vi "test-AsyncMessageWithReplyWithErrorWithGlobalVariable.vi"(8 "error in (no error)":errorcluster, 11 "TestCase in":refnum<class "testcase-CSMMessage.lvclass">) -> (0 "error out":errorcluster, 3 "TestCase out":refnum<class "testcase-CSMMessage.lvclass">)   [LabVIEW 2017, in "testcase-CSMMessage.lvclass"]
uses:
  testcase-CSMMessage.lvclass
  C:/Program Files (x86)/National Instruments/LabVIEW 2017/vi.lib/addons/_JKI Toolkits/VI Tester/TestCase.llb/TestCase.lvclass
  src/user.lib/_NEVSTOP/Communicable State Machine(CSM)/Communicable State Machine.lvlib
  CSM/Global-TestcaseCSM.vi
  CSM/CSM-Testcase.lvlib
  <vilib>/addons/_JKI Toolkits/VI Tester/TestCase.llb/TestCase.lvclass
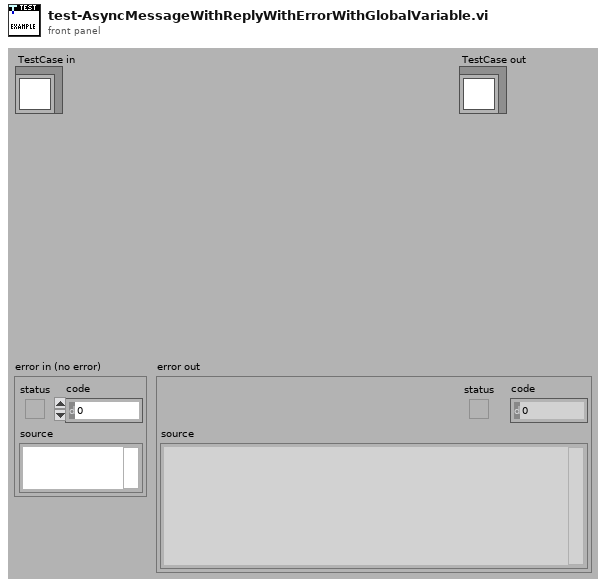
[diagram p1: front panel]
types:
  T1 = cluster{"Arguments":string, "Response":string, "error":errorcluster}
  T2 = cluster{"status":bool, "code":bool, "source":bool}
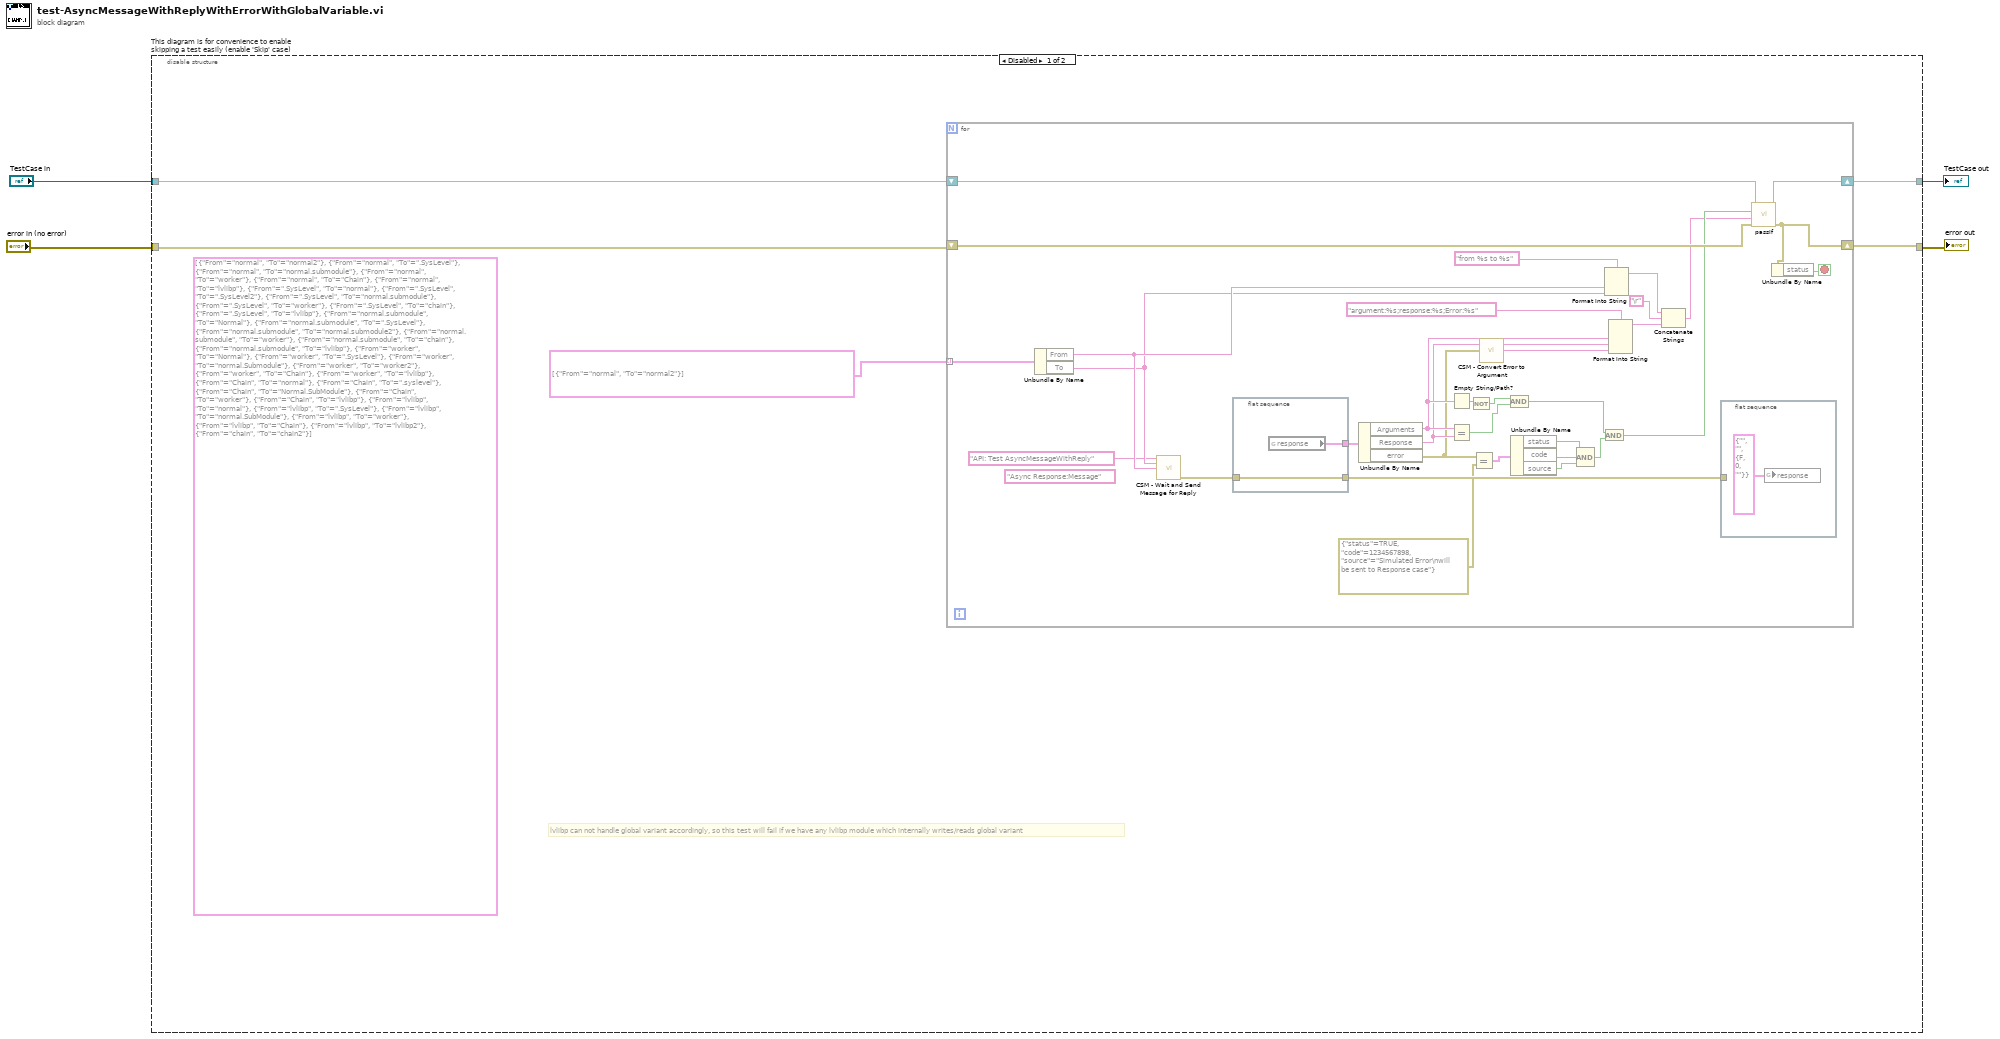
[diagram p0: block diagram]
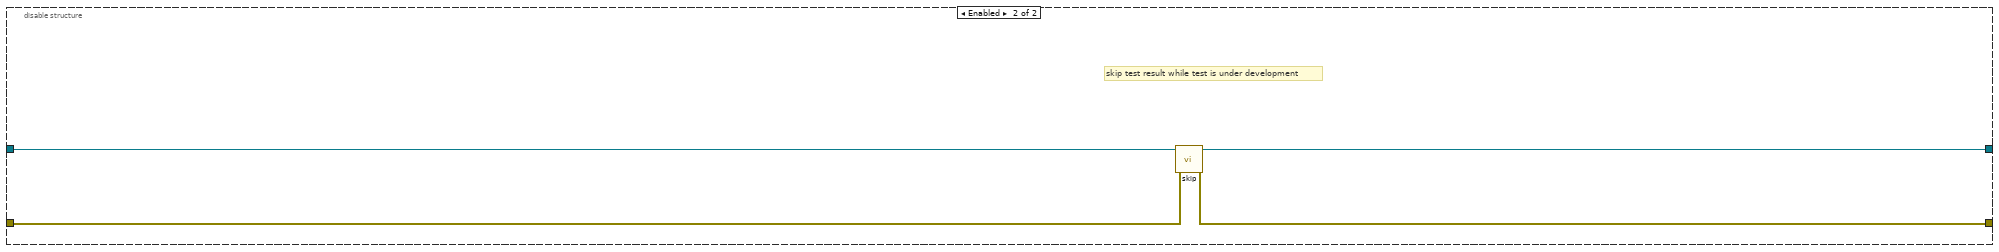
[diagram p2: hidden frame]
diagram:
  n1 = disable-structure "This diagram is for convenience to enable skipping a test easily (enable 'Skip' case)" shown="Disabled" {
    disable-tunnel: "TestCase in" -> [w9 w49]
    disable-tunnel: [w8 w47] -> w1
    disable-tunnel: [w6 w48] -> w3
    disable-tunnel: "error in (no error)" -> [w7 w46]
    frame Disabled {
      (unwired) cluster{"From":string, "To":string}[] [{"From"="normal", "To"="normal2"}, {"From"="normal", "To"=".SysLevel"}, {"From"="normal", "To"="normal.submodule"}, {"From"="normal", "To"="worker"}, {"From"="normal", "To"="Chain"}, {"From"="normal", "To"="lvlibp"}, {"From"=".SysLevel", "To"="normal"}, {"From"=".SysLevel", "To"=".SysLevel2"}, {"From"=".SysLevel", "To"="normal.submodule"}, {"From"=".SysLevel", "To"="worker"}, {"From"=".SysLevel", "To"="chain"}, {"From"=".SysLevel", "To"="lvlibp"}, {"From"="normal.submodule", "To"="Normal"}, {"From"="normal.submodule", "To"=".SysLevel"}, {"From"="normal.submodule", "To"="normal.submodule2"}, {"From"="normal.submodule", "To"="worker"}, {"From"="normal.submodule", "To"="chain"}, {"From"="normal.submodule", "To"="lvlibp"}, {"From"="worker", "To"="Normal"}, {"From"="worker", "To"=".SysLevel"}, {"From"="worker", "To"="normal.Submodule"}, {"From"="worker", "To"="worker2"}, {"From"="worker", "To"="Chain"}, {"From"="worker", "To"="lvlibp"}, {"From"="Chain", "To"="normal"}, {"From"="Chain", "To"=".syslevel"}, {"From"="Chain", "To"="Normal.SubModule"}, {"From"="Chain", "To"="worker"}, {"From"="Chain", "To"="lvlibp"}, {"From"="lvlibp", "To"="normal"}, {"From"="lvlibp", "To"=".SysLevel"}, {"From"="lvlibp", "To"="normal.SubModule"}, {"From"="lvlibp", "To"="worker"}, {"From"="lvlibp", "To"="Chain"}, {"From"="lvlibp", "To"="lvlibp2"}, {"From"="chain", "To"="chain2"}]
      # "lvlibp can not handle global variant accordingly, so this test will fail if we have any lvlibp module which internally writes/reads global variant"
      n2 = for {
        tunnel: cluster{"From":string, "To":string}[] [{"From"="normal", "To"="normal2"}] -> [w38] mode=indexing
        shift-right: [w41] -> w8
        shift-left: w9 -> [w42]
        shift-right: [w21] -> w6
        shift-left: w7 -> [w40]
        stop <- w20 stop-if-true
        (unwired) "Async Response:Message" ("State")
        n3 = Unbundle By Name(w38) -> ("From"=w19:string, "To"=w18:string)
        n4 = call "CSM - Wait and Send Message for Reply.vi"("State"="API: Test AsyncMessageWithReply", "Arguments (\"\")"=w18, "Target Module"=w19) -> ("error out"=w22:errorcluster)  [unwired: 10 in, 2 out]
        n5 = flat-sequence {
          tunnel: w22 -> [w44]
          tunnel: [w45] -> w24
          tunnel: [w44] -> w23
          frame #0 {
            n6 = global read "Global-TestcaseCSM.vi" "response"() -> (w45:T1)
          }
        }
        n7 = Unbundle By Name(w24) -> ("Arguments"=w32:string, "Response"=w31:string, "error"=w17:errorcluster)
        n8 = Empty String/Path?(string/path=w32) -> (empty?=w36:bool)
        n9 = Equal?(x=w32, y=w31) -> (x = y?=w34:bool)
        n10 = Not(x=w36) -> (.not. x?=w35:bool)
        n11 = Equal?(x=w17, y=errorcluster {"status"=TRUE, "code"=1234567898, "source"="Simulated Error\nwill be sent to Response case"} ("error out")) -> (x = y?=w13:T2)
        n12 = call "CSM - Convert Error to Argument.vi"("Error"=w17) -> ("Argument"=w30:string)  [unwired: 4 in]
        n13 = And(x=w35, y=w34) -> (x .and. y?=w33:bool)
        n14 = Unbundle By Name(w13) -> ("status"=w15:bool, "code"=w14:bool, "source"=w12:bool)
        n15 = Compound Arithmetic op=AND(w15, w14, w12) -> (w11:bool)
        n16 = And(x=w33, y=w11) -> (x .and. y?=w39:bool)
        n17 = Format Into String(format string="from %s to %s", w19, w18) -> (resulting string=w26:string)  [unwired: 2 in, 1 out]
        n18 = Format Into String(format string="argument:%s;response:%s;Error:%s", w32, w31, w30) -> (resulting string=w29:string)  [unwired: 2 in, 1 out]
        n19 = Concatenate Strings(w26, "\r", w29) -> (w27:string)
        n20 = flat-sequence {
          tunnel: w23 -> [_]
          frame #0 {
            n21 = global write "Global-TestcaseCSM.vi" "response"(T1 {"Arguments"="", "Response"="", "error"={"status"=FALSE, "code"=0, "source"=""}} ("response")) -> ()
          }
        }
        n22 = call-dynamic "passIf.vi"("error in (no error)"=w40, "message (\"\")"=w27, "pass"=w39, "TestCase in"=w42) -> ("error out"=w21:errorcluster, "TestCase out"=w41:refnum<class "testcase-CSMMessage.lvclass">)  [unwired: 6 in]
        n23 = Unbundle By Name(w21) -> ("status"=w20:bool)
      }
    }
    frame Enabled {
      # "skip test result while test is under development"
      n24 = call <vilib>:"skip.vi"("error in (no error)"=w46, "TestCase in"=w49) -> ("error out"=w48:errorcluster, "TestCase out"=w47:refnum<class "testcase-CSMMessage.lvclass">)  [unwired: 8 in]
    }
  }
  "error out" <- w3
  "TestCase out" <- w1
